vi "ROISettings.vi"(5 "ROISizes":u16[](array[numeric]), 6 "SizeEnum":string[](array[string]), 7 "ImgArray":u32[][](graph)=array640x480[307200 elements], 8 "ROIHeight":u16, 9 "ROIWidth":u16, 10 "ROIYOffset":u16, 11 "ROIXOffset":u16) -> (0 "ROIHeightOUT":u16, 1 "ROIWidthOUT":u16, 2 "ROIYOffsetOUT":u16, 3 "ROIXOffsetOUT":u16, 4 "SizesOUT":i32(ring) items=["2.6\" x 2.6\" (20 x 20 pixels)", "5.2\" x 5.2\" (40 x 40 pixels)", "7.7\" x 7.7\" (60 x 60 pixels)", "10.3\" x 10.3\" (80 x 80 pixels)", "12.9\" x 12.9\" (100 x 100 pixels)", "20.6\" x 20.6\" (160 x 160 pixels)"])   [LabVIEW 2019]
panel:
  out "size(s)":i32[](array[numeric])
  in  "Ring":i32(ring) items=["2.6\" x 2.6\"", "5.2\" x 5.2\"", "7.7\" x 7.7\"", "10.3\" x 10.3\"", "12.9\" x 12.9\"", "20.6\" x 20.6\""]
  in  "cancel":bool
  in  "accept":bool
  out "subimg":u32[][](graph)
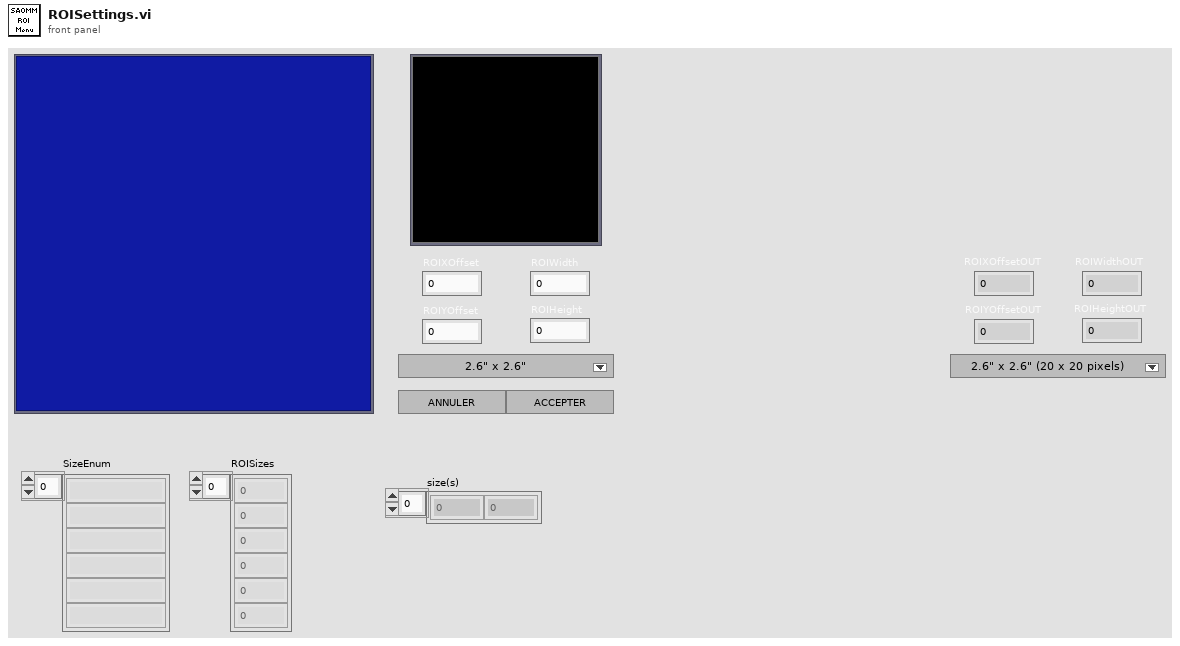
[diagram p1: front panel]
types:
  T1 = typedef "LVPoint32TypeDef.ctl" = cluster{"Horizontal":i32, "Vertical":i32}
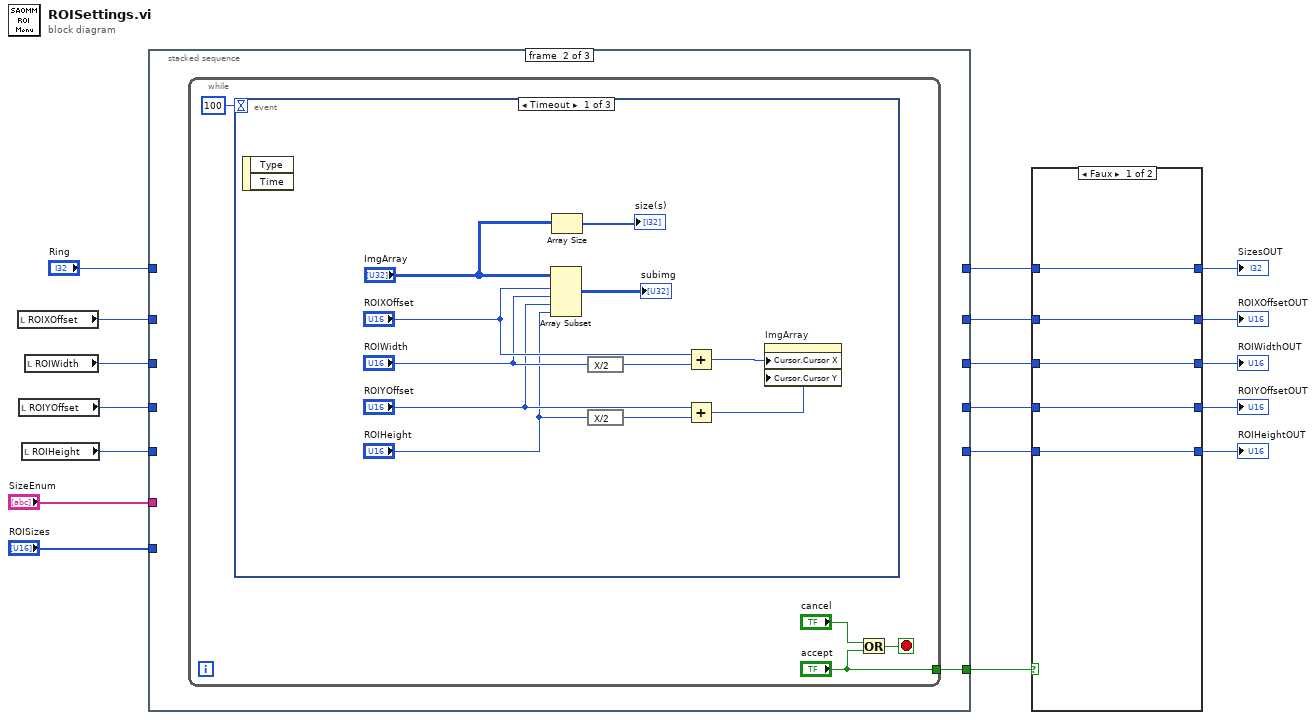
[diagram p0: block diagram]
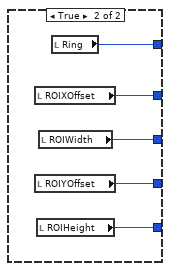
[diagram p2: hidden frame]
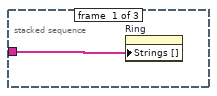
[diagram p3: hidden frame]
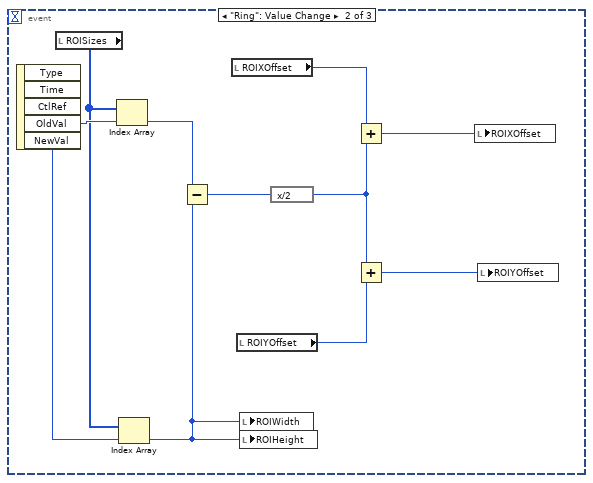
[diagram p4: hidden frame]
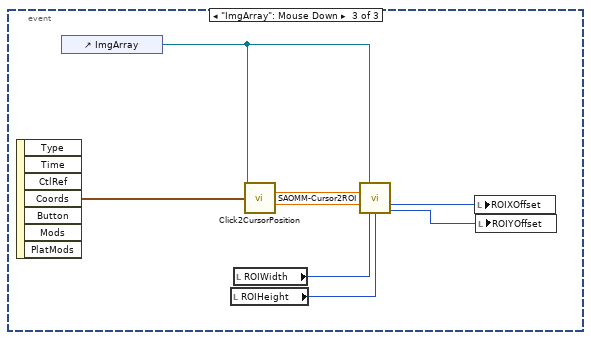
[diagram p5: hidden frame]
diagram:
  n1 = local read "ROIXOffset"() -> (w15:u16)
  n2 = local read "ROIYOffset"() -> (w13:u16)
  n3 = local read "ROIHeight"() -> (w12:u16)
  n4 = local read "ROIWidth"() -> (w14:u16)
  n5 = stacked-sequence {
    tunnel: "SizeEnum" -> [w19 _ _]
    tunnel: "ROISizes" -> [_ _ _]
    tunnel: [_ w20 _] -> w16
    tunnel: w15 -> [_ _ w59]
    tunnel: w14 -> [_ _ w58]
    tunnel: w13 -> [_ _ w57]
    tunnel: w12 -> [_ _ w56]
    tunnel: [_ _ w59] -> w11
    tunnel: [_ _ w58] -> w10
    tunnel: [_ _ w57] -> w9
    tunnel: [_ _ w56] -> w8
    tunnel: "Ring" -> [_ _ w55]
    tunnel: [_ _ w55] -> w5
    frame #0 {
      n6 = property on="Ring" class="MDér (strict)"("Strings []"=w19) -> ()  [unwired: 2 in, 2 out]
    }
    frame #1 {
      n7 = while {
        tunnel: ["accept"] -> w20
        stop <- w24 stop-if-true
        n8 = event shown="[0] Timeout" {
          selector: _ -> [_ _ _]
          dyn-events: _ -> [_ _ _]
          timeout: 100 -> [_ _ _]
          event Timeout {
            n9 = event-data() -> ()  [unwired: 1 in, 2 out]
            n10 = Array Subset(array="ImgArray", index (row)="ROIXOffset", length (row)="ROIWidth", index (col)="ROIYOffset", length (col)="ROIHeight") -> (→"subimg":u32[][])
            n11 = Array Size(array="ImgArray") -> (size(s)=→"size(s)":i32[])
            n12 = expression code="X/2"("ROIWidth") -> (w31:u16)
            n13 = expression code="X/2"("ROIHeight") -> (w30:u16)
            n14 = Add(x="ROIXOffset", y=w31) -> (x+y=w33:u16)
            n15 = Add(x="ROIYOffset", y=w30) -> (x+y=w32:u16)
            n16 = property on="ImgArray" class="GraphInt (strict)"("Cursor.Cursor X"=w33, "Cursor.Cursor Y"=w32) -> ()  [unwired: 2 in, 2 out]
          }
          event "Ring": Value Change {
            n17 = event-data() -> ("OldVal"=w46:i32, "NewVal"=w45:i32)  [unwired: 1 in, 3 out]
            n18 = local read "ROISizes"() -> (w44:u16[])
            n19 = Index Array(array=w44, index=w46) -> (element=w43:u16)
            n20 = Index Array(array=w44, index=w45) -> (element=w42:u16)
            n21 = Subtract(x=w43, y=w42) -> (x-y=w41:u16)
            n22 = local read "ROIXOffset"() -> (w40:u16)
            n23 = local read "ROIYOffset"() -> (w37:u16)
            n24 = local write "ROIWidth"(w42) -> ()
            n25 = local write "ROIHeight"(w42) -> ()
            n26 = expression code="x/2"(w41) -> (w38:u16)
            n27 = Add(x=w40, y=w38) -> (x+y=w39:u16)
            n28 = Add(x=w38, y=w37) -> (x+y=w36:u16)
            n29 = local write "ROIXOffset"(w39) -> ()
            n30 = local write "ROIYOffset"(w36) -> ()
          }
          event "ImgArray": Mouse Down {
            n31 = event-data() -> ("Coords"=w49:T1)  [unwired: 1 in, 6 out]
            n32 = control-ref of="ImgArray"() -> (w50:refnum<vi>)
            n33 = local read "ROIHeight"() -> (w51:u16)
            n34 = local read "ROIWidth"() -> (w52:u16)
            n35 = call "Click2CursorPosition.vi"("reference"=w50, "ClickPosition"=w49) -> ("CursorX"=w53:dbl, "CursorY"=w54:dbl)  [unwired: 12 in]
            n36 = call "SAOMM-Cursor2ROI.vi"("ImgRef"=w50, "CursorX"=w53, "CursorY"=w54, "ROIWidth"=w52, "ROIHeight"=w51) -> ("ROIXOffset"=w48:u16, "ROIYOffset"=w47:u16)  [unwired: 7 in, 2 out]
            n37 = local write "ROIXOffset"(w48) -> ()
            n38 = local write "ROIYOffset"(w47) -> ()
          }
        }
        n39 = Or(x="cancel", y="accept") -> (x .or. y?=w24:bool)
      }
    }
    frame #2 {
    }
  }
  n40 = case shown="Faux" w16 {
    tunnel: w11 -> [w60 _]
    tunnel: w10 -> [w61 _]
    tunnel: w9 -> [w62 _]
    tunnel: w8 -> [w63 _]
    tunnel: [w64 w69] -> w7
    tunnel: w5 -> [w64 _]
    tunnel: [w63 w65] -> w4
    tunnel: [w62 w66] -> w3
    tunnel: [w61 w67] -> w2
    tunnel: [w60 w68] -> w1
    frame False {
    }
    frame True {
      n41 = local read "ROIXOffset"() -> (w68:u16)
      n42 = local read "ROIYOffset"() -> (w66:u16)
      n43 = local read "ROIHeight"() -> (w65:u16)
      n44 = local read "ROIWidth"() -> (w67:u16)
      n45 = local read "Ring"() -> (w69:i32)
    }
  }
  "SizesOUT" <- w7
  "ROIYOffsetOUT" <- w3
  "ROIXOffsetOUT" <- w1
  "ROIHeightOUT" <- w4
  "ROIWidthOUT" <- w2
